vi "Lean Back angle Calc.vi"(10 "z":dbl, 11 "r1":dbl) -> (2 "Elbow Angle":dbl, 3 "Shoulder Angle":dbl)   [LabVIEW 2018]
uses:
  Arm Constants.vi
panel:
  out "temp":dbl
  out "eint":dbl
  out "erad":dbl
  out "trad":dbl
  out "prad":dbl
  out "y":dbl
  out "alpha":dbl
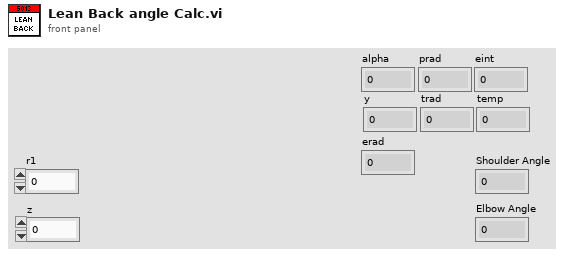
[diagram p1: front panel]
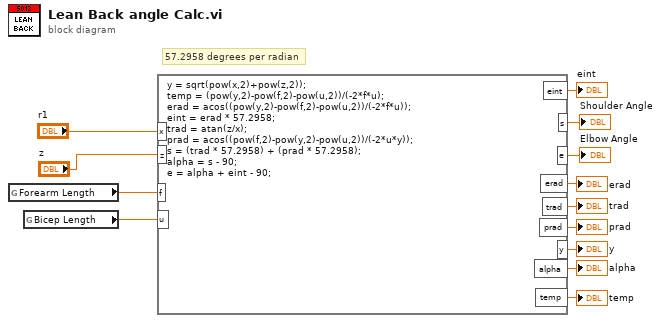
[diagram p0: block diagram]
diagram:
  # "57.2958 degrees per radian"
  n1 = global read "Arm Constants.vi" "Forearm Length"() -> (w9:dbl)
  n2 = global read "Arm Constants.vi" "Bicep Length"() -> (w8:dbl)
  n3 = formula code="y = sqrt(pow(x,2)+pow(z,2));\ntemp = (pow(y,2)-pow(f,2)-pow(u,2))/(-2*f*u);\nerad = acos((pow(y,2)-pow(f,2)-pow(u,2))/(-2*f*u));\neint = erad * 57.2958;\ntrad = atan(z/x);\nprad = acos((pow(f,2)-pow(y,2)-pow(u,2))/(-2*u*y));\ns = (trad * 57.2958) + (prad * 57.2958);\nalpha = s - 90;\ne = alpha + eint - 90;"("x"="r1", "z"="z", "f"=w9, "u"=w8) -> ("s"=→"Shoulder Angle":dbl, "e"=→"Elbow Angle":dbl, "erad"=→"erad":dbl, "trad"=→"trad":dbl, "prad"=→"prad":dbl, "y"=→"y":dbl, "eint"=→"eint":dbl, "alpha"=→"alpha":dbl, "temp"=→"temp":dbl)
